vi "GPSPressCANRead.vi"(8 "Error In":errorcluster, 10 "NodeID":u8, 11 "ObjHandle In":u32) -> (0 "Error Out":errorcluster, 2 "Pressure":sgl, 3 "ObjHandle Out":u32)   [LabVIEW 2019]
panel:
  out "error out":errorcluster
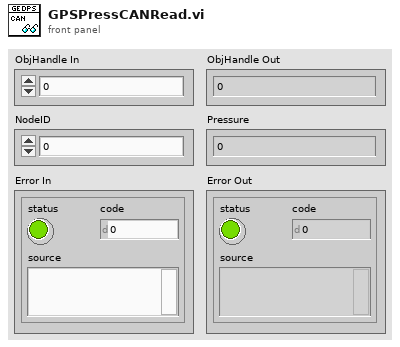
[diagram p1: front panel]
types:
  T1 = enum16{"big-endian, network order", "native, host order", "little-endian"}
  T2 = typedef "xobjhandle.ctl" = u32
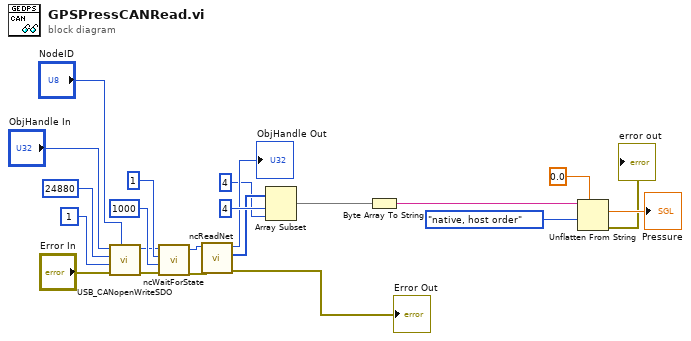
[diagram p0: block diagram]
diagram:
  n1 = call "USB_CANopenWriteSDO.vi"("Node ID"="NodeID", "error in"="Error In", "Sub Index"=u8 1 ("object sub-index (0)"), "Index"=u16 24880 ("object index"), "ObjHandle in"="ObjHandle In") -> ("error out"=w18:errorcluster, "ObjHandle out"=w20:T2)  [unwired: 5 in]
  n2 = call <vilib>:"ncWaitForState.vi"("Error in"=w18, "Timeout"=u32 1000, "DesiredState"=u32 1, "ObjHandle in"=w20) -> ("Error out"=w1:errorcluster, "ObjHandle out"=w19:T2)  [unwired: 1 out]
  n3 = call <vilib>:"ncReadNet.vi"("ObjHandle in"=w19, "Error in"=w1) -> ("ObjHandle out"=→"ObjHandle Out":T2, "Data"=w15:u8[], "Error out"=→"Error Out":errorcluster)  [unwired: 2 in, 4 out]
  n4 = Array Subset(array=w15, index=4, length=4) -> (w9:u8[])
  n5 = Byte Array To String(unsigned byte array=w9) -> (string=w17:string)
  n6 = Unflatten From String(type=sgl 0.0, binary string=w17, byte order (0:big-endian, network order)=T1."native, host order") -> (value=→"Pressure":sgl, error out=→"error out":errorcluster)  [unwired: 2 in, 1 out]
